vi "ListVIs.vi"(7 "Scope":T1, 8 "error in":errorcluster, 9 "RepoRoot":path, 10 "Remote Branch to Compare":string, 11 "Folder Path":path) -> (0 "error out":errorcluster, 3 "VIs":path[](array[path])=[path "C:/Users/pauloneill/SCC/Orion/LabVIEW/CICD/CLIOperations/AnalyzeVIs/Create Directory if Necessary.vi", path "C:/Users/pauloneill/SCC/Orion/LabVIEW/CICD/CLIOperations/AnalyzeVIs/GetHelp.vi", path "C:/Users/pauloneill/SCC/Orion/LabVIEW/CICD/CLIOperations/AnalyzeVIs/ParseArguments.vi", path "C:/Users/pauloneill/SCC/Orion/LabVIEW/CICD/CLIOperations/AnalyzeVIs/ParseArgumentsCore.vi", path "C:/Users/pauloneill/SCC/Orion/LabVIEW/CICD/CLIOperations/AnalyzeVIs/ParseResult.vi", path "C:/Users/pauloneill/SCC/Orion/LabVIEW/CICD/CLIOperations/AnalyzeVIs/RunOperation.vi", path "C:/Users/pauloneill/SCC/Orion/LabVIEW/CICD/CLIOperations/AnalyzeVIs/VerifyArguments.vi", path "C:/Users/pauloneill/SCC/Orion/LabVIEW/CICD/CLIOperations/ApplyVIPC/GetHelp.vi", path "C:/Users/pauloneill/SCC/Orion/LabVIEW/CICD/CLIOperations/ApplyVIPC/ParseArguments.vi", path "C:/Users/pauloneill/SCC/Orion/LabVIEW/CICD/CLIOperations/ApplyVIPC/RunOperation.vi", path "C:/Users/pauloneill/SCC/Orion/LabVIEW/CICD/CLIOperations/ApplyVIPC/Utilities/ValidateVIPCPath.vi", path "C:/Users/pauloneill/SCC/Orion/LabVIEW/CICD/CLIOperations/ApplyVIPC/Utilities/VerifyArguments.vi", path "C:/Users/pauloneill/SCC/Orion/LabVIEW/CICD/CLIOperations/Build/ParseArguments.vi", path "C:/Users/pauloneill/SCC/Orion/LabVIEW/CICD/CLIOperations/Build/RunOperation.vi", path "C:/Users/pauloneill/SCC/Orion/LabVIEW/CICD/CLIOperations/ClearCompileCache.vi", path "C:/Users/pauloneill/SCC/Orion/LabVIEW/CICD/CLIOperations/ClearCompileCache/GetHelp.vi", path "C:/Users/pauloneill/SCC/Orion/LabVIEW/CICD/CLIOperations/ClearCompileCache/ParseArguments.vi", path "C:/Users/pauloneill/SCC/Orion/LabVIEW/CICD/CLIOperations/ClearCompileCache/RunOperation.vi", path "C:/Users/pauloneill/SCC/Orion/LabVIEW/CICD/CLIOperations/ClearCompileCache/Utilities/ClearCompileCache--function.vi", path "C:/Users/pauloneill/SCC/Orion/LabVIEW/CICD/CLIOperations/CompiledCodeSeparated.vi", path "C:/Users/pauloneill/SCC/Orion/LabVIEW/CICD/GCLI/ApplyVIPC.vi", path "C:/Users/pauloneill/SCC/Orion/LabVIEW/CICD/GCLI/RunUnitTest.vi", path "C:/Users/pauloneill/SCC/Orion/LabVIEW/CICD/GCLI/VIAnalyzer.vi", path "C:/Users/pauloneill/SCC/Orion/LabVIEW/CICD/GCLI/VIPBuild.vi", path "C:/Users/pauloneill/SCC/Orion/LabVIEW/CICD/Helpers/AnalyzeVI--function.vi", path "C:/Users/pauloneill/SCC/Orion/LabVIEW/CICD/Helpers/ApplyVIPC--function.vi", path "C:/Users/pauloneill/SCC/Orion/LabVIEW/CICD/Helpers/Build--function.vi", path "C:/Users/pauloneill/SCC/Orion/LabVIEW/CICD/Helpers/VIAnalyzer--function.vi", path "C:/Users/pauloneill/SCC/Orion/LabVIEW/CICD/Private/GITChangedFiles.vi", path "C:/Users/pauloneill/SCC/Orion/LabVIEW/CICD/Private/GITGetRoot.vi", path "C:/Users/pauloneill/SCC/Orion/LabVIEW/CICD/Private/ListVIs.vi", path "C:/Users/pauloneill/SCC/Orion/LabVIEW/CICD/Test/GIT Paths.vi"])   [LabVIEW 2020, in "CICD.lvlib"]
doc: "List the VIs in the repo or folder depending on the scope selected. Scope can be \"ChangedFiles\", \"Folder\", or \"All\".\n\"ChangedFiles\" and \"All\" require GIT. Default is \"ChangedFiles\"."
uses:
  CICD.lvlib
  <vilib>/ErrorRing/Error Ring.xnode
  <vilib>/Utility/error.llb/Error Cluster From Error Code.vi
  Scope--enum.ctl
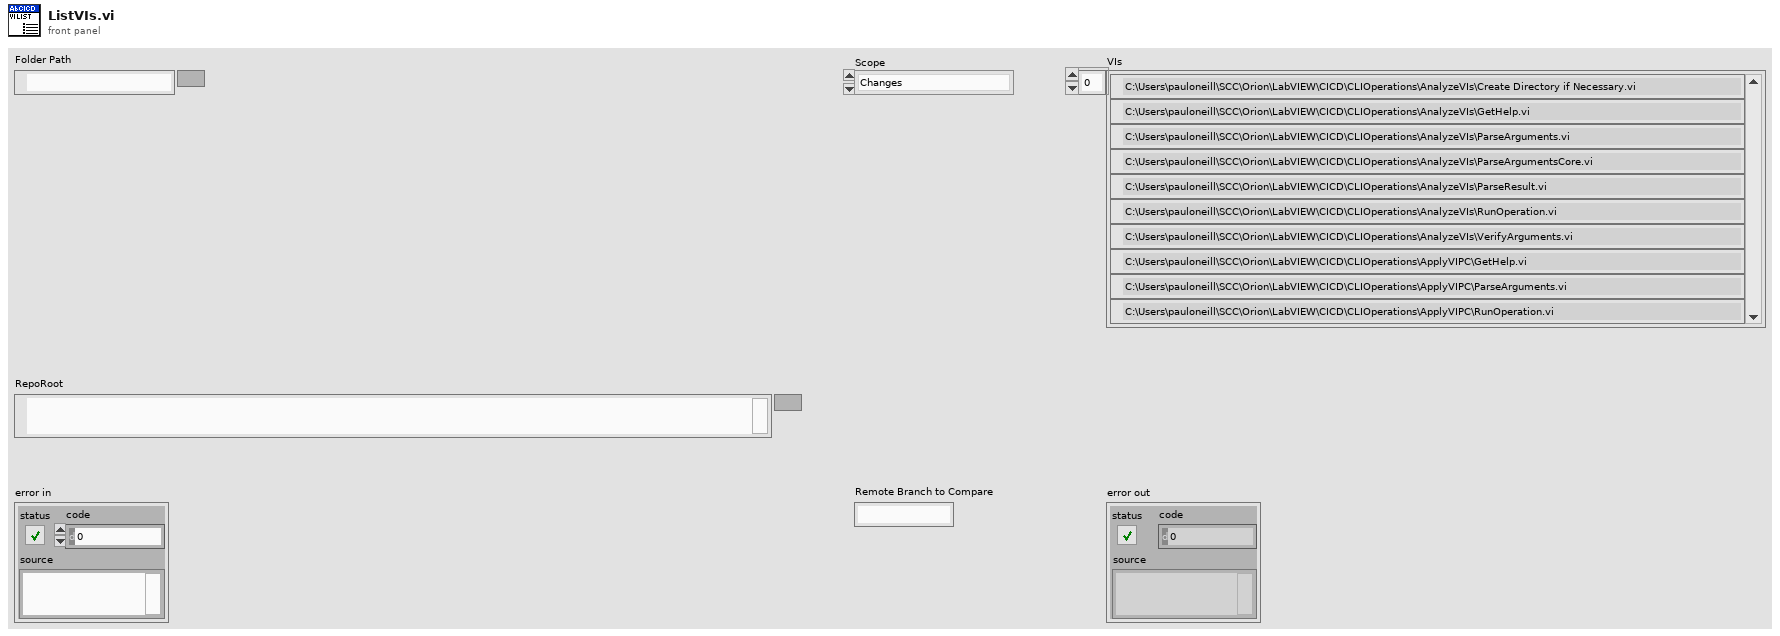
[diagram p1: front panel]
types:
  T1 = typedef "CICD.lvlib/Scope--enum.ctl" = enum16{"Changes", "All", "Folder"}
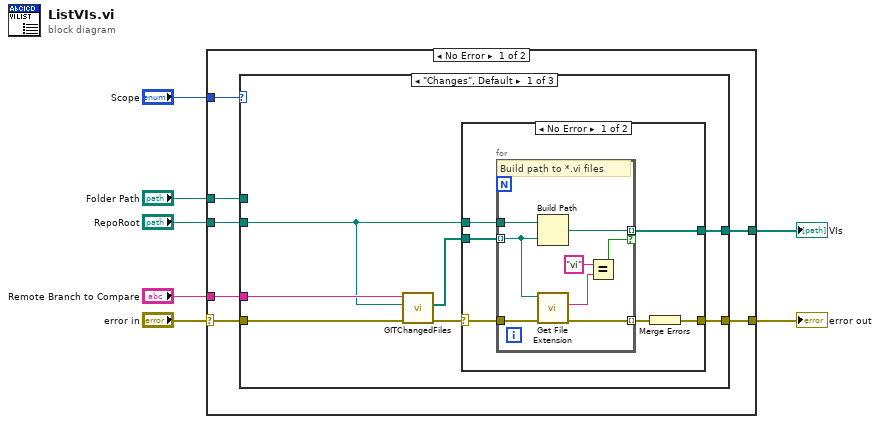
[diagram p0: block diagram]
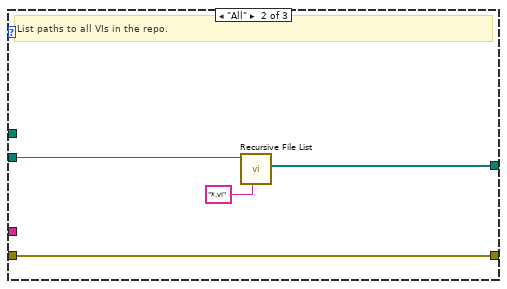
[diagram p3: hidden frame]
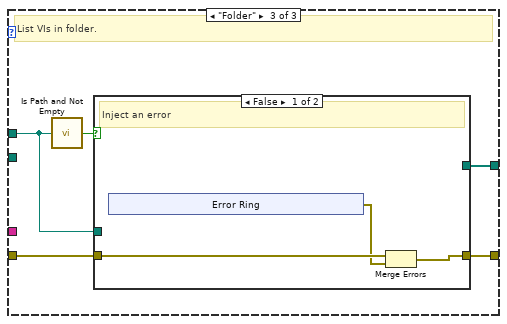
[diagram p4: hidden frame]
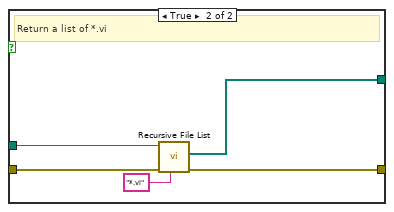
[diagram p5: hidden frame]
diagram:
  n1 = case shown="No Error" "error in" {
    selector: "error in" -> [w13 w58]
    tunnel: [w14 w58] -> w7
    tunnel: "Scope" -> [w12 _]
    tunnel: "Remote Branch to Compare" -> [w11 _]
    tunnel: [w10 _] -> w3
    tunnel: "Folder Path" -> [w9 _]
    tunnel: "RepoRoot" -> [w8 _]
    frame No Error {
      n2 = case shown="\"Changes\", Default" w12 {
        tunnel: w13 -> [w21 w40 w45]
        tunnel: [w20 w40 w44] -> w14
        tunnel: w11 -> [w18 _ _]
        tunnel: [w16 w38 w43] -> w10
        tunnel: w9 -> [_ _ w42]
        tunnel: w8 -> [w15 w37 _]
        frame "Changes", Default {
          n3 = call "GITChangedFiles.vi"("error in"=w21, "RepoRoot"=w15, "Remote Branch to Compare"=w18) -> ("error out"=w19:errorcluster, "Files Changed"=w17:path[])  [unwired: 7 in]
          n4 = case shown="No Error" w19 {
            selector: w19 -> [w26 w36]
            tunnel: w15 -> [w25 _]
            tunnel: w17 -> [w24 _]
            tunnel: [w23 _] -> w16
            tunnel: [w27 w36] -> w20
            frame No Error {
              n5 = for {
                tunnel: w25 -> [w33]
                tunnel: w24 -> [w31] mode=indexing
                tunnel: [w32] -> w23 mode=indexing if=w28
                tunnel: w26 -> [w35]
                tunnel: [w34] -> w22 mode=indexing
                # "Build path to *.vi files"
                n6 = Build Path(base path=w33, name or relative path=w31) -> (appended path=w32:path)
                n7 = call <vilib>:"Get File Extension.vi"("error in (no error)"=w35, "file"=w31) -> ("error out"=w34:errorcluster, "lowercase file extension"=w30:string)  [unwired: 5 in, 3 out]
                n8 = Equal?(x="vi", y=w30) -> (x = y?=w28:bool)
              }
              n9 = Merge Errors(w22) -> (w27:errorcluster)
            }
            frame Error {
            }
          }
        }
        frame "All" {
          # "List paths to all VIs in the repo."
          n10 = call <vilib>:"Recursive File List.vi"("pattern"="*.vi", "Folder Path"=w37) -> ("All Files in Dir"=w38:path[])  [unwired: 5 in, 4 out]
        }
        frame "Folder" {
          # "List VIs in folder."
          n11 = call <vilib>:"Is Path and Not Empty.vi"("path"=w42) -> ("Is Path and Not Empty?"=w41:bool)  [unwired: 4 in]
          n12 = case shown="False" w41 {
            tunnel: w45 -> [w48 w57]
            tunnel: [w47 w56] -> w44
            tunnel: [_ w54] -> w43
            tunnel: w42 -> [_ w53]
            frame False {
              # "Inject an error"
              n13 = xnode "Error Ring"() -> ("error out"=w46:errorcluster)
              n14 = Merge Errors(w48, w46) -> (w47:errorcluster)
            }
            frame True {
              # "Return a list of *.vi"
              n15 = call <vilib>:"Recursive File List.vi"("pattern"="*.vi", "error in (no error)"=w57, "Folder Path"=w53) -> ("error out"=w56:errorcluster, "All Files in Dir"=w54:path[])  [unwired: 4 in, 3 out]
            }
          }
        }
      }
    }
    frame Error {
    }
  }
  "error out" <- w7
  "VIs" <- w3
